vi "Bounds.vi"(1 "XRef":refnum<vi>, 2 "State In":T2) -> (0 "Bounds":cluster{"Width":T1, "Height":T1})   [LabVIEW 2018, in "OpenG Reorder Array.xnode"]
uses:
  OpenG Reorder Array.xnode
  State.ctl
  <vilib>/XNodeSupport/XNodeInt.ctl
  <vilib>/XNodeSupport/NI_XNodeSupport.lvlib
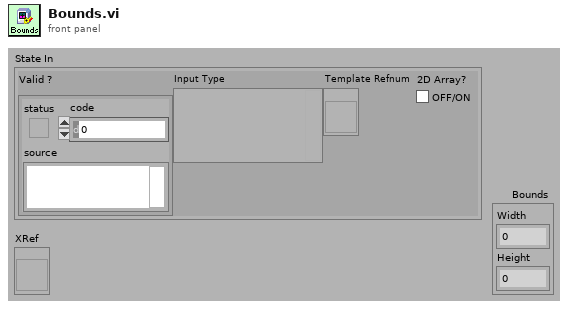
[diagram p1: front panel]
types:
  T1 = typedef "NI_XNodeSupport.lvlib/XNodeInt.ctl" = i32
  T2 = typedef "OpenG Reorder Array.xnode/State.ctl" = cluster{"Valid ?":errorcluster, "Input Type":variant, "Template Refnum":refnum<vi>, "2D Array?":bool}
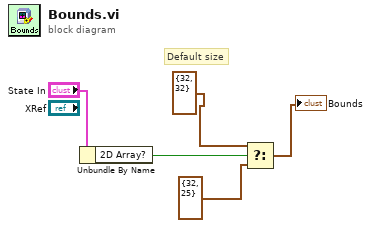
[diagram p0: block diagram]
diagram:
  # "Default size"
  n1 = Unbundle By Name("State In") -> ("2D Array?"=w4:bool)
  n2 = Select(t=cluster{"Width":T1, "Height":T1} {"Width"=32, "Height"=32} ("Bounds"), s=w4, f=cluster{"Width":T1, "Height":T1} {"Width"=32, "Height"=25} ("Bounds")) -> (s? t:f=→"Bounds":cluster{"Width":T1, "Height":T1})
